vi "close.vi"(11 "Experience ID":string) -> (0 "error out":errorcluster)   [LabVIEW 2020]
panel:
  # "Close"
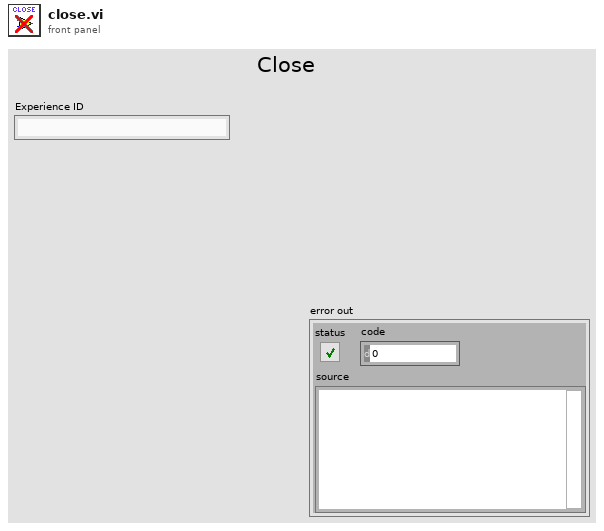
[diagram p1: front panel]
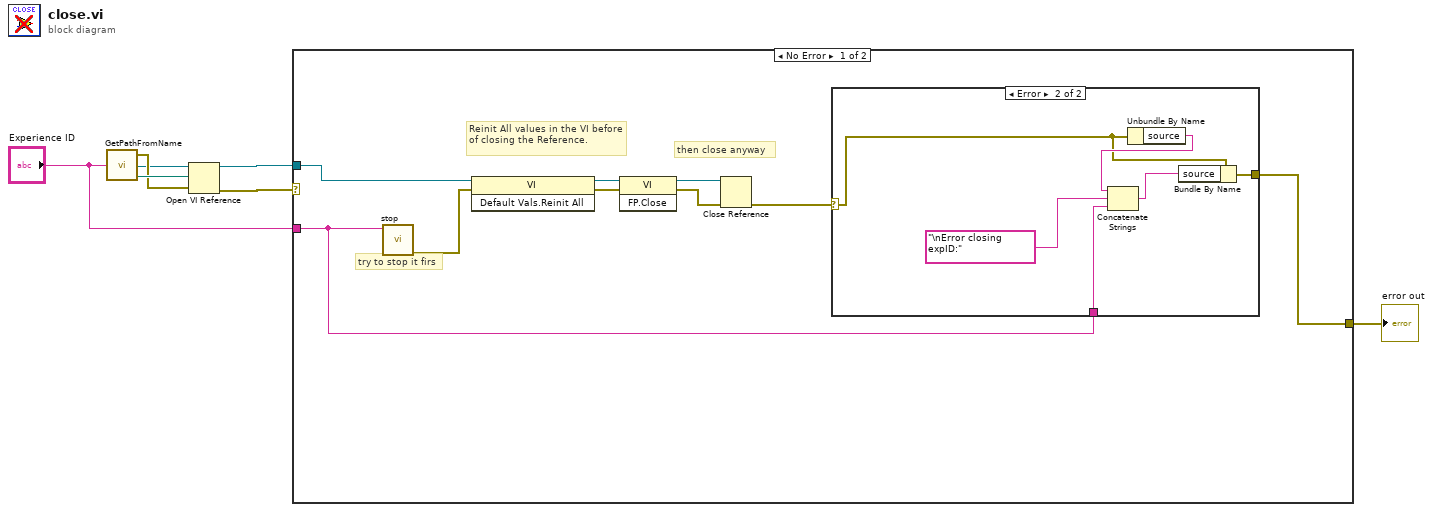
[diagram p0: block diagram]
diagram:
  n1 = call "GetPathFromName.vi"("Experience ID"="Experience ID") -> ("VI_Path"=w7:path, "application reference"=w1:refnum<vi>, "Error out"=w6:errorcluster)  [unwired: 2 in]
  n2 = Open VI Reference(application reference (local)=w1, vi path=w7, error in (no error)=w6) -> (vi reference=w3:refnum<vi>, error out=w4:errorcluster)  [unwired: 3 out]
  n3 = case shown="No Error" w4 {
    selector: w4 -> [_ w24]
    tunnel: [w8 w24] -> w5
    tunnel: w3 -> [w11 _]
    tunnel: "Experience ID" -> [w9 _]
    frame No Error {
      # "try to stop it firs"
      # "then close anyway"
      # "Reinit All values in the VI before of closing the Reference."
      n4 = call "stop.vi"("Experience ID"=w9) -> ("error out"=w12:errorcluster)  [unwired: 10 in]
      n5 = invoke class="VI" method="Default Vals.Reinit All"(reference=w11, error in=w12) -> (reference out=w16:refnum<vi>, error out=w15:errorcluster)  [unwired: 1 in, 1 out]
      n6 = invoke class="VI" method="FP.Close"(reference=w16, error in=w15) -> (reference out=w14:refnum<vi>, error out=w13:errorcluster)  [unwired: 1 in, 1 out]
      n7 = Close Reference(reference=w14, error in (no error)=w13) -> (error out=w10:errorcluster)
      n8 = case shown="Error" w10 {
        selector: w10 -> [w17 w19]
        tunnel: [w17 w23] -> w8
        tunnel: w9 -> [_ w18]
        frame No Error {
        }
        frame Error {
          n9 = Unbundle By Name(w19) -> ("source"=w22:string)
          n10 = Concatenate Strings(w22, "\nError closing expID:" ("FailDescriptor"), w18) -> (w21:string)
          n11 = Bundle By Name(cluster=w19, "source"=w21) -> (w23:errorcluster)
        }
      }
    }
    frame Error {
    }
  }
  "error out" <- w5
